vi "RunOperation.vi"(10 "Inputs":string[](array[string]), 11 "LUnitCLI in":refnum<class "LUnitCLI.lvclass">) -> (1 "Output/Failure":string, 2 "CLI Process Return Code":i32, 3 "LUnitCLI out":refnum<class "LUnitCLI.lvclass">)   [LabVIEW 2020, in "LUnitCLI.lvclass"]
uses:
  LUnitCLI.lvclass
  LUnitCLI.lvclass/LUnitCLI.ctl
  Execution API/Execution API.lvclass
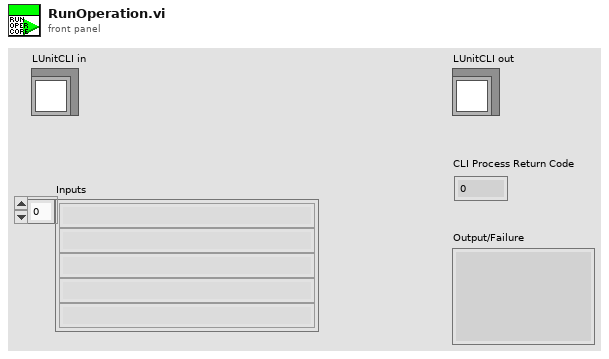
[diagram p1: front panel]
types:
  T1 = cluster{"Event Registration Refnum":refnum<event-registration>, "Event Registration Refnum":refnum<event-registration>}
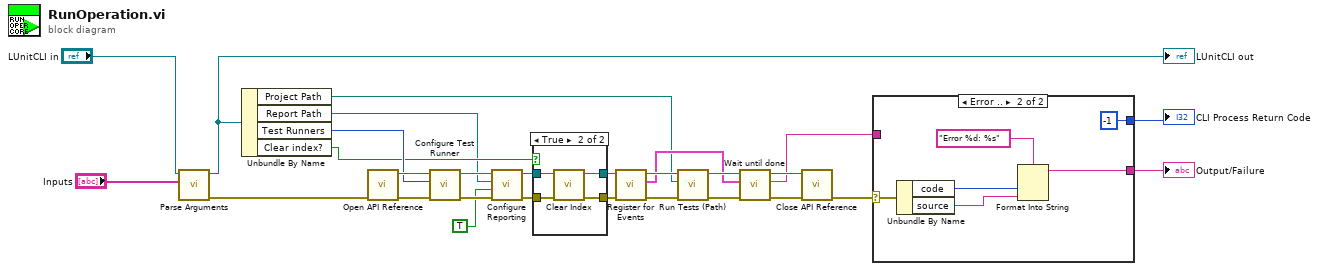
[diagram p0: block diagram]
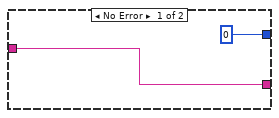
[diagram p3: hidden frame]
diagram:
  n1 = call "Parse Arguments.vi"("Inputs"="Inputs", "LUnitCLI in"="LUnitCLI in") -> ("error out"=w3:errorcluster, "LUnitCLI out"=w24:refnum<class "LUnitCLI.lvclass">)  [unwired: 8 in]
  "LUnitCLI out" <- w24
  n2 = Unbundle By Name(w24) -> ("Project Path"=w1:path, "Report Path"=w7:path, "Test Runners"=w9:i32, "Clear index?"=w8:bool)
  n3 = call "Open API Reference.vi"("error in (no error)"=w3) -> ("error out"=w22:errorcluster, "Execution API out"=w23:refnum<class "Execution API.lvclass">)  [unwired: 9 in]
  n4 = call "Configure Test Runner.vi"("error in (no error)"=w22, "Number of Test Runners"=w9, "Execution API In"=w23) -> ("error out"=w20:errorcluster, "Execution API Out"=w21:refnum<class "Execution API.lvclass">)  [unwired: 7 in]
  n5 = call "Configure Reporting.vi"("error in (no error)"=w20, "Autogenerate?"=TRUE, "Path"=w7, "Execution API In"=w21) -> ("error out"=w18:errorcluster, "Execution API Out"=w19:refnum<class "Execution API.lvclass">)  [unwired: 6 in]
  n6 = case shown="True" w8 {
    tunnel: w19 -> [w30 w34]
    tunnel: w18 -> [w29 w33]
    tunnel: [w30 w32] -> w17
    tunnel: [w29 w31] -> w16
    frame False {
    }
    frame True {
      n7 = call "Clear Index.vi"("error in (no error)"=w33, "Execution API In"=w34) -> ("error out"=w31:errorcluster, "Execution API Out"=w32:refnum<class "Execution API.lvclass">)  [unwired: 8 in]
    }
  }
  n8 = call "Register for Events.vi"("error in (no error)"=w16, "Execution API In"=w17) -> ("error out"=w14:errorcluster, "Result Events Registration"=w5:T1, "Execution API Out"=w15:refnum<class "Execution API.lvclass">)  [unwired: 7 in]
  n9 = call "Run Tests (Path).vi"("error in (no error)"=w14, "Project or Class Path"=w1, "Execution API In"=w15) -> ("error out"=w12:errorcluster, "Execution API Out"=w13:refnum<class "Execution API.lvclass">)  [unwired: 7 in]
  n10 = call "Wait until done.vi"("error in (no error)"=w12, "Result Events"=w5, "Execution API In"=w13) -> ("error out"=w10:errorcluster, "Output"=w4:string, "Execution API Out"=w11:refnum<class "Execution API.lvclass">)  [unwired: 6 in]
  n11 = call "Close API Reference.vi"("error in (no error)"=w10, "Execution API in"=w11) -> ("error out"=w2:errorcluster)  [unwired: 9 in]
  n12 = case shown="Error .." w2 {
    selector: w2 -> [_ w41]
    tunnel: [w36 w37] -> w28
    tunnel: w4 -> [w36 _]
    tunnel: [0 ("CLI Process Return Code") -1 ("CLI Process Return Code")] -> w27
    frame No Error {
    }
    frame Error {
      n13 = Unbundle By Name(w41) -> ("code"=w40:i32, "source"=w39:string)
      n14 = Format Into String(format string="Error %d: %s", w40, w39) -> (resulting string=w37:string)  [unwired: 2 in, 1 out]
    }
  }
  "CLI Process Return Code" <- w27
  "Output/Failure" <- w28
